vi "GetModuleInfo.vi"(0 "reference in":refnum<class "DQMHModuleNode.lvclass">, 5 "error in (no error)":errorcluster) -> (7 "Description":string, 9 "ModuleUnmodified":path, 10 "Template":string, 11 "Events(string)":string, 12 "Base class.bounds":T1 {"height" format="%.2f"; "width" format="%.2f"; "y" format="%.2f"; "x" format="%.2f"}, 13 "Events((string)":string, 14 "reference out":refnum<class "DQMHModuleNode.lvclass">, 15 "ModuleName":string, 16 "InternalData":string[](array[string]), 17 "Events":string[](array[string]), 18 "ModulePath":path, 19 "error out":errorcluster)   [LabVIEW 2016, in "DQMHModuleNode.lvclass"]
uses:
  <resource>/Framework/Providers/Open_GDS/UML/DQMHModuleNode_class/DQMHModuleNode.lvclass
  C:/Program Files (x86)/National Instruments/LabVIEW 2016/resource/Framework/Providers/Open_GDS/UML/RectangularNode_class/RectangularNode.lvclass
  <resource>/Framework/Providers/Open_GDS/UML/General/Rectangle/Rectangle Rectangle2D.ctl
  <resource>/Framework/Providers/Open_GDS/UML/MultiLineString_class/MultiLineString.lvclass
  <resource>/Framework/Providers/Open_GDS/UML/RectangularNode_class/RectangularNode.lvclass
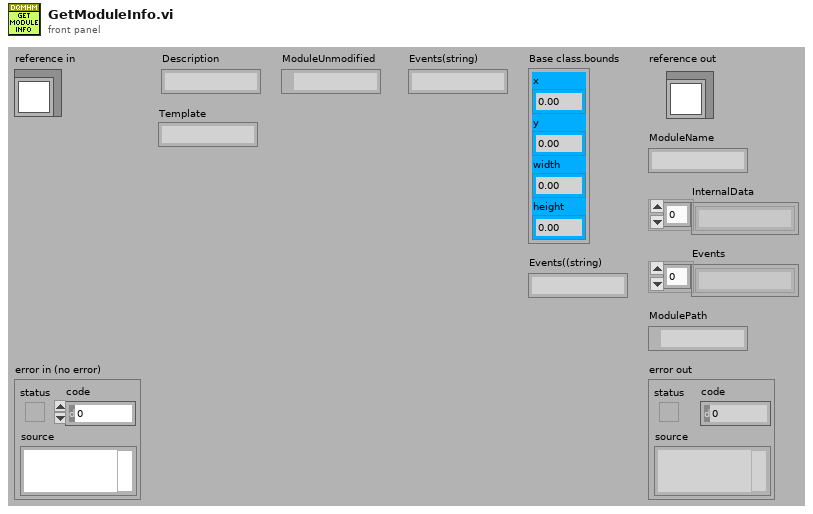
[diagram p1: front panel]
types:
  T1 = typedef "Rectangle Rectangle2D.ctl" = cluster{"x":dbl, "y":dbl, "width":dbl, "height":dbl}
  T2 = typedef "DQMHModuleNode.lvclass/ObjectAttributes.ctl" = cluster{"DescriptionHeight":dbl, "InternalDataHeight":dbl, "EventsHeight":dbl, "Name":refnum<class "MultiLineString.lvclass">, "Description":refnum<class "MultiLineString.lvclass">, "InternalData":refnum<class "MultiLineString.lvclass">, "Events":refnum<class "MultiLineString.lvclass">, "showDescription":bool, "showInternalData":bool, "showEvents":bool, "DEFAULT_ROUNDING":i32, "DEFAULT_WIDTH":i32, "DEFAULT_HEIGHT":i32, "ClassPath":path, "Template":string, "Icon":u8[][]}
  T3 = typedef "RectangularNode.lvclass/ObjectAttributes.ctl" = cluster{"bounds":T1}
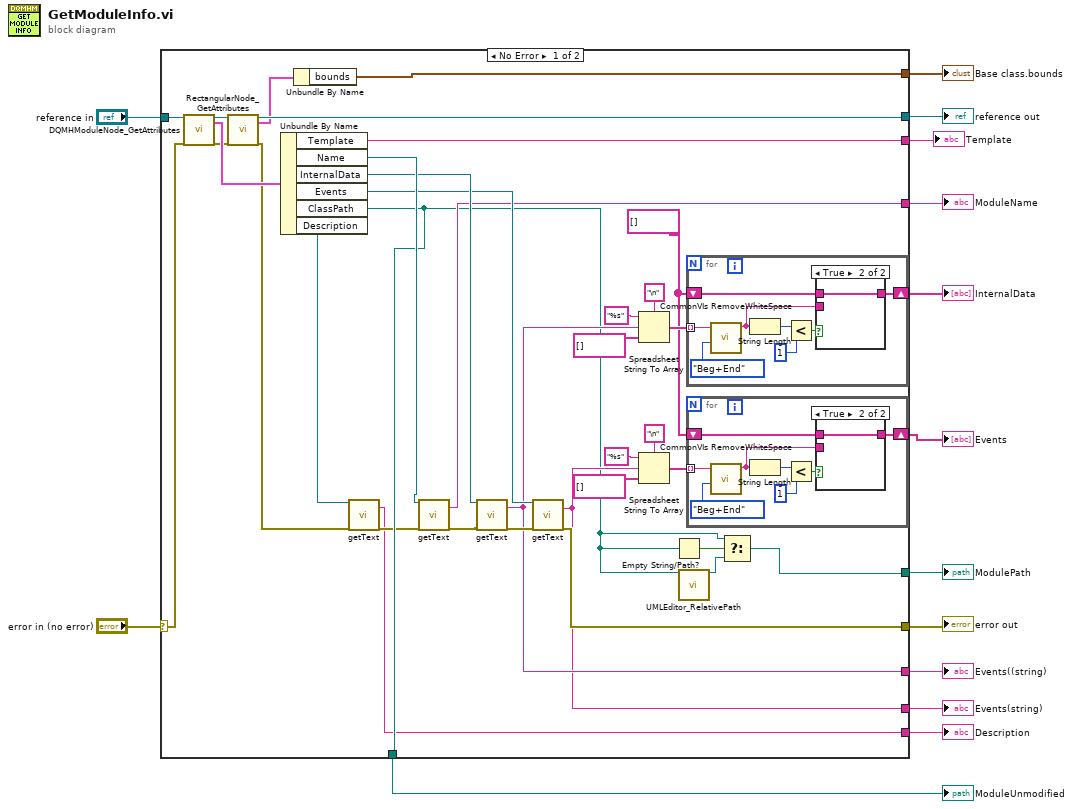
[diagram p0: block diagram]
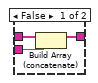
[diagram p2: hidden frame]
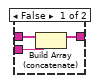
[diagram p3: hidden frame]
diagram:
  n1 = case shown="No Error" "error in (no error)" {
    selector: "error in (no error)" -> [w51 w76]
    tunnel: "reference in" -> [w50 w77]
    tunnel: [w47 w76] -> w12
    tunnel: [w21 w77] -> w11
    tunnel: [w43 _] -> w10
    tunnel: [w38 _] -> w9
    tunnel: [w33 _] -> w8
    tunnel: [w26 _] -> w7
    tunnel: [w31 _] -> w6
    tunnel: [w30 _] -> w5
    tunnel: [w28 _] -> w4
    tunnel: [w25 _] -> w3
    tunnel: [w16 _] -> w2
    tunnel: [w15 _] -> w1
    frame No Error {
      w32 = string[] []
      n2 = call <resource>:"DQMHModuleNode_GetAttributes.vi"("reference in"=w50, "error in (no error)"=w51) -> ("reference out"=w23:refnum<class "DQMHModuleNode.lvclass">, "Data"=w24:T2, "error out"=w22:errorcluster)  [unwired: 1 in, 14 out]
      n3 = call <resource>:"RectangularNode_GetAttributes.vi"("reference in"=w23, "error in (no error)"=w22) -> ("reference out"=w21:refnum<class "DQMHModuleNode.lvclass">, "Data"=w20:T3, "error out"=w19:errorcluster)  [unwired: 14 in, 1 out]
      n4 = Unbundle By Name(w24) -> ("Template"=w15:string, "Name"=w46:refnum<class "MultiLineString.lvclass">, "InternalData"=w45:refnum<class "MultiLineString.lvclass">, "Events"=w44:refnum<class "MultiLineString.lvclass">, "ClassPath"=w28:path, "Description"=w17:refnum<class "MultiLineString.lvclass">)
      n5 = Unbundle By Name(w20) -> ("bounds"=w25:T1)
      n6 = call-dynamic "getText.vi"("reference"=w17, "error in (no error)"=w19) -> ("text"=w16:string, "error out"=w18:errorcluster)  [unwired: 16 out]
      n7 = call-dynamic "getText.vi"("reference"=w46, "error in (no error)"=w18) -> ("text"=w43:string, "error out"=w49:errorcluster)  [unwired: 16 out]
      n8 = call-dynamic "getText.vi"("reference"=w45, "error in (no error)"=w49) -> ("text"=w31:string, "error out"=w48:errorcluster)  [unwired: 16 out]
      n9 = call-dynamic "getText.vi"("reference"=w44, "error in (no error)"=w48) -> ("text"=w30:string, "error out"=w47:errorcluster)  [unwired: 16 out]
      n10 = Spreadsheet String To Array(delimiter (Tab)="\n", format string="%s", spreadsheet string=w31, array type (2D Dbl)=string[] []) -> (array=w39:string[])
      n11 = Spreadsheet String To Array(delimiter (Tab)="\n", format string="%s", spreadsheet string=w30, array type (2D Dbl)=string[] []) -> (array=w37:string[])
      n12 = Empty String/Path?(string/path=w28) -> (empty?=w29:bool)
      n13 = call <resource>:"UMLEditor_RelativePath.vi"("Path In"=w28) -> ("ConvertToAbsolutePath(If possible)"=w27:path)  [unwired: 1 in, 17 out]
      n14 = for {
        tunnel: w39 -> [w71] mode=indexing
        shift-right: [w64] -> w38
        shift-left: w32 -> [w66]
        n15 = call <resource>:"CommonVIs RemoveWhiteSpace.vi"("Remove from"=enum16{"Begining", "End", "Beg+End", "All"}."Beg+End", "String in"=w71) -> ("String out"=w65:string)  [unwired: 2 in, 3 out]
        n16 = String Length(string=w65) -> (length=w69:i32)
        n17 = Less?(x=w69, y=1) -> (x < y?=w67:bool)
        n18 = case shown="True" w67 {
          tunnel: w66 -> [w74 w75]
          tunnel: w65 -> [w73 _]
          tunnel: [w72 w75] -> w64
          frame False {
            n19 = Build Array (concatenate)(w74, w73) -> (w72:string[])
          }
          frame True {
          }
        }
      }
      n20 = for {
        tunnel: w37 -> [w59] mode=indexing
        shift-right: [w52] -> w33
        shift-left: w32 -> [w54]
        n21 = call <resource>:"CommonVIs RemoveWhiteSpace.vi"("Remove from"=enum16{"Begining", "End", "Beg+End", "All"}."Beg+End", "String in"=w59) -> ("String out"=w53:string)  [unwired: 2 in, 3 out]
        n22 = String Length(string=w53) -> (length=w57:i32)
        n23 = Less?(x=w57, y=1) -> (x < y?=w55:bool)
        n24 = case shown="True" w55 {
          tunnel: w54 -> [w62 w63]
          tunnel: w53 -> [w61 _]
          tunnel: [w60 w63] -> w52
          frame False {
            n25 = Build Array (concatenate)(w62, w61) -> (w60:string[])
          }
          frame True {
          }
        }
      }
      n26 = Select(t=w28, s=w29, f=w27) -> (s? t:f=w26:path)
    }
    frame Error {
    }
  }
  "reference out" <- w11
  "error out" <- w12
  "ModuleName" <- w10
  "InternalData" <- w9
  "Events" <- w8
  "ModulePath" <- w7
  "Events((string)" <- w6
  "Events(string)" <- w5
  "ModuleUnmodified" <- w4
  "Base class.bounds" <- w3
  "Description" <- w2
  "Template" <- w1
